vi "rs3 process frame.vi"(8 "error in (no error)":errorcluster, 10 "Frame":u64, 11 "Processing Block":u64) -> (0 "error out":errorcluster, 2 "frame out":u64, 3 "error process frame":u64)   [LabVIEW 2018, in "libRealSense3.lvlib"]
doc: "Provides timestamp"
uses:
  libRealSense3.lvlib
  realsense2.dll
panel:
  # "RS3 Process Frame"
  # "(C) Intel Corp.,  AGJ"
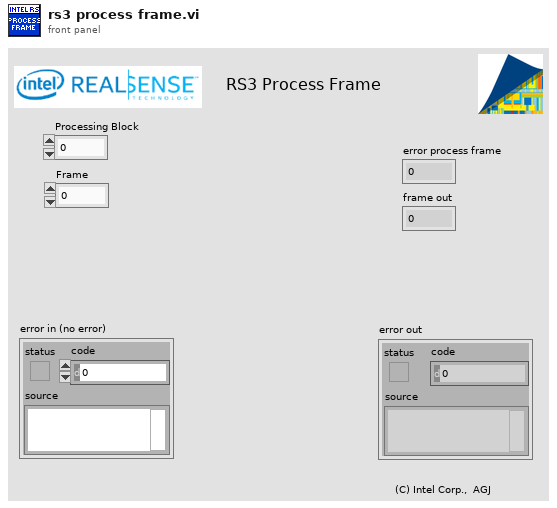
[diagram p1: front panel]
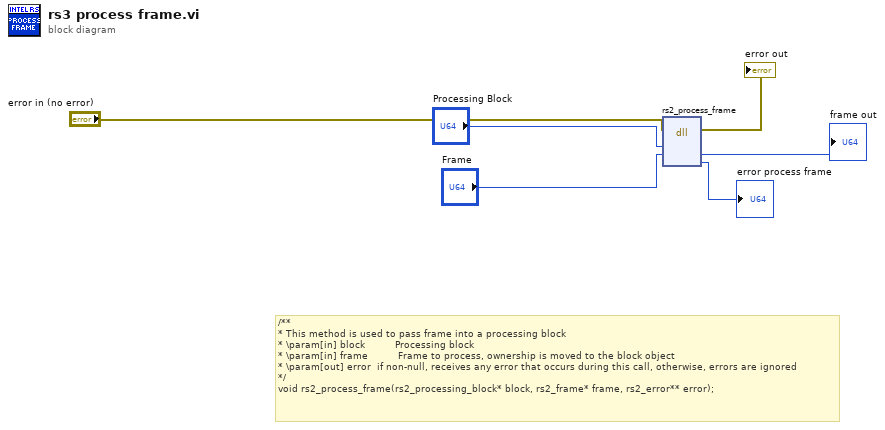
[diagram p0: block diagram]
diagram:
  # "/**\n* This method is used to pass frame into a processing block\n* \\param[in] block          Processing block\n* \\param[in] frame          Frame to process, ownership is moved to the block object\n* \\param[out] error  if non-null, receives any error that occurs during this call, otherwise, errors are ignored\n*/\nvoid rs2_process_frame(rs2_processing_block* block, rs2_frame* frame, rs2_error** error);"
  n1 = dll-call lib="C:/Users/aaron.jencks/Documents/GitHub/emerson_seed_object_detection/LabVIEW/Projects/Paul's Video Viewer/Classes/Realsense Cam/realsense_wrapper_api/realsense2.dll" fn="rs2_process_frame"(error in="error in (no error)", "processing block"="Processing Block", "frame"="Frame") -> (error out=→"error out":errorcluster, "frame"=→"frame out":u64, "error"=→"error process frame":u64)  [unwired: 5 in, 1 out]
